vi "FGV_OEE_reference_selector.vi"(7 "options":T1, 8 "error_in":errorcluster, 11 "input":variant) -> (0 "error_out":errorcluster, 3 "output":variant)   [LabVIEW 2019]
uses:
  FGV_OEE_reference_selector.ctl
  OEE_reference_selecotr_references.ctl
  _misc/AULocalize/SubVIs/Get Localized Phrase Compact Interface 0D.vi
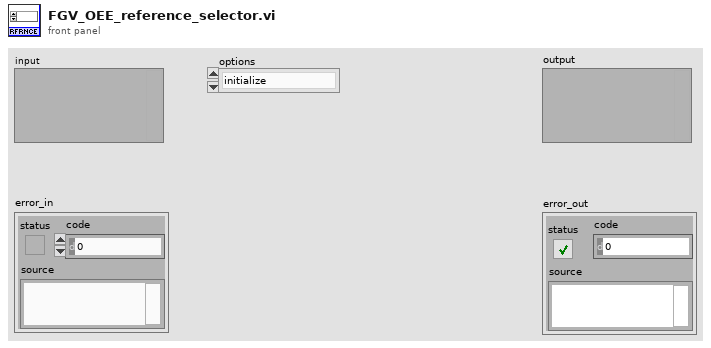
[diagram p1: front panel]
types:
  T1 = typedef "FGV_OEE_reference_selector.ctl" = enum16{"initialize", "set_values", "enable", "disable", "disable_gray", "get_reference_list", "get_active_reference"}
  T2 = typedef "OEE_reference_selecotr_references.ctl" = cluster{"reference_list":string[], "reference_selector":refnum<vi>, "reload_reference_list":refnum<vi>, "toggle_pulses":refnum<vi>}
  T3 = enum8{"Enabled", "Disabled", "Disabled and Grayed Out"}
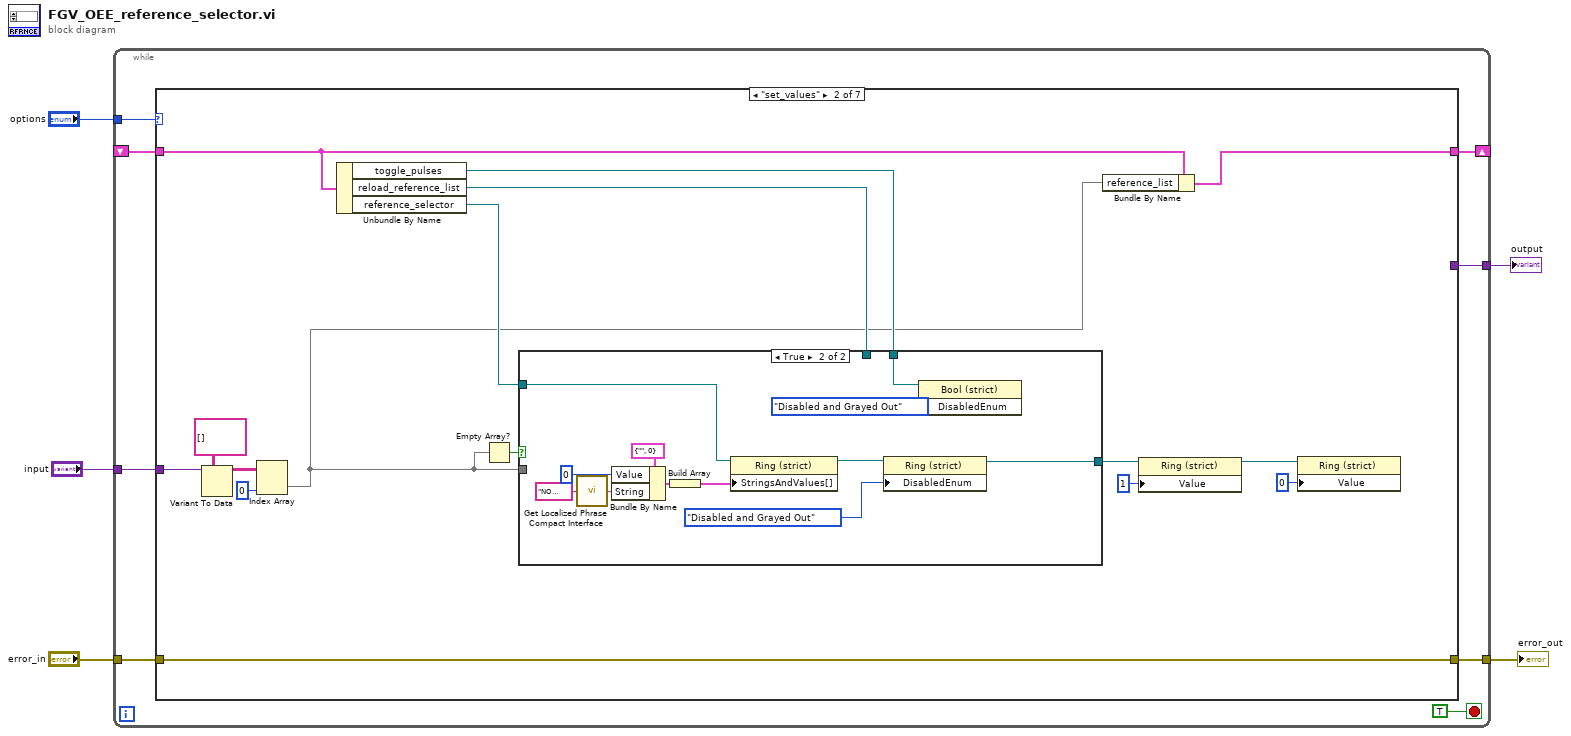
[diagram p0: block diagram]
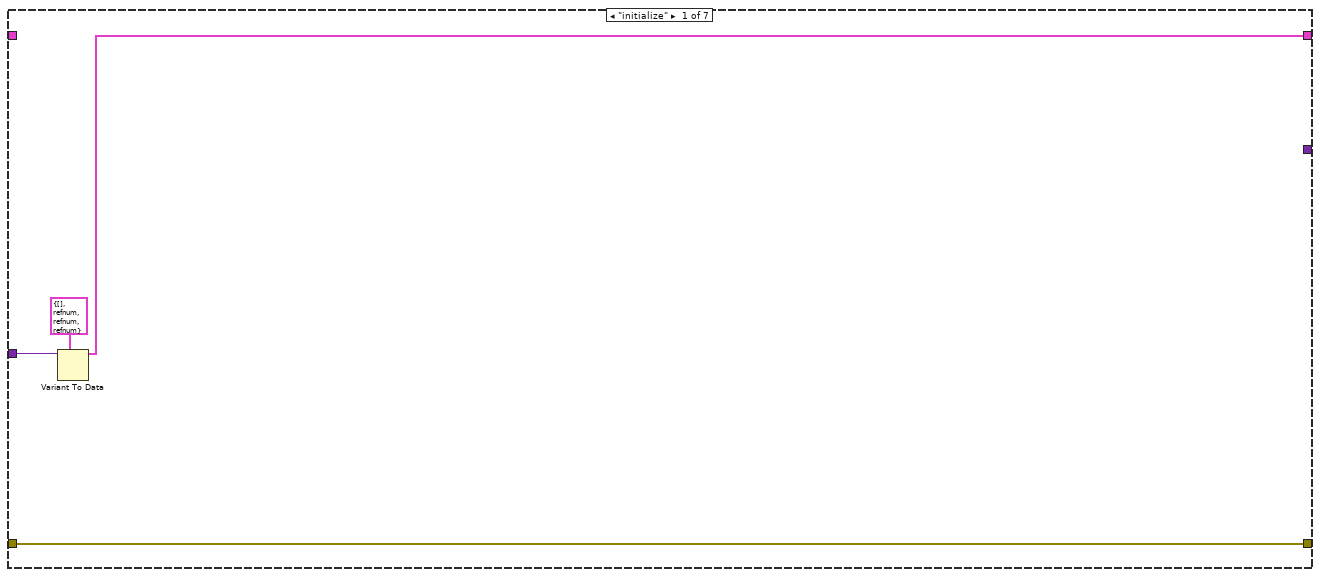
[diagram p2: hidden frame]
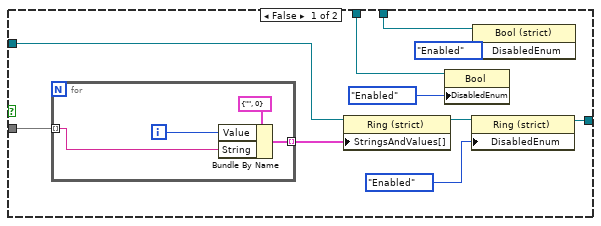
[diagram p3: hidden frame]
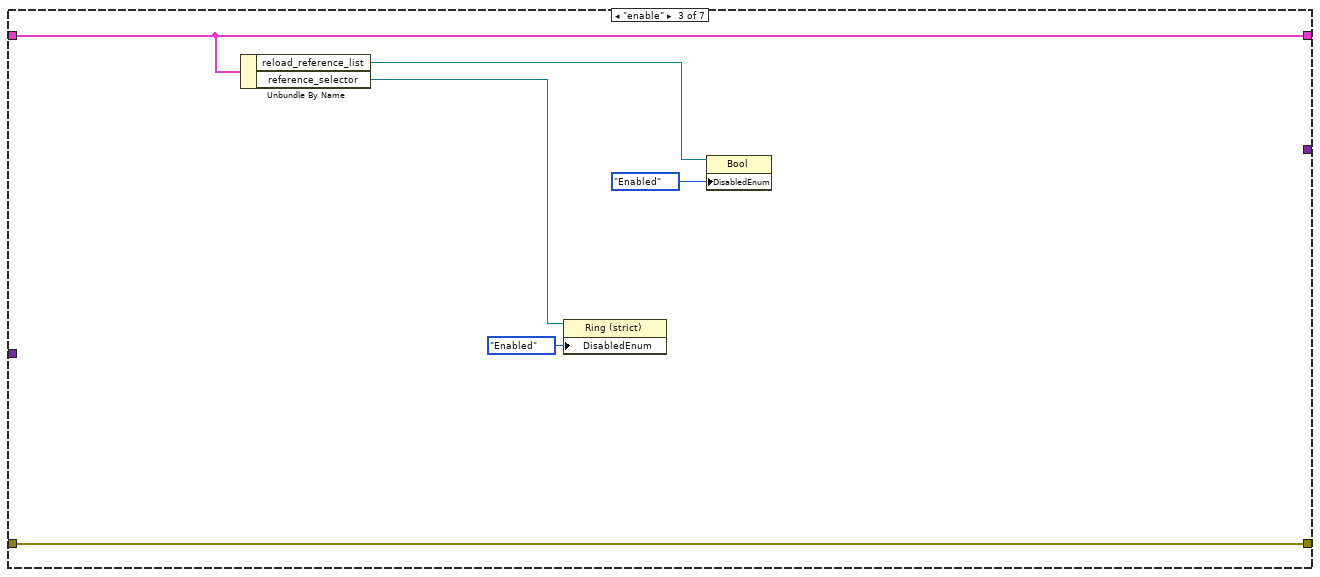
[diagram p4: hidden frame]
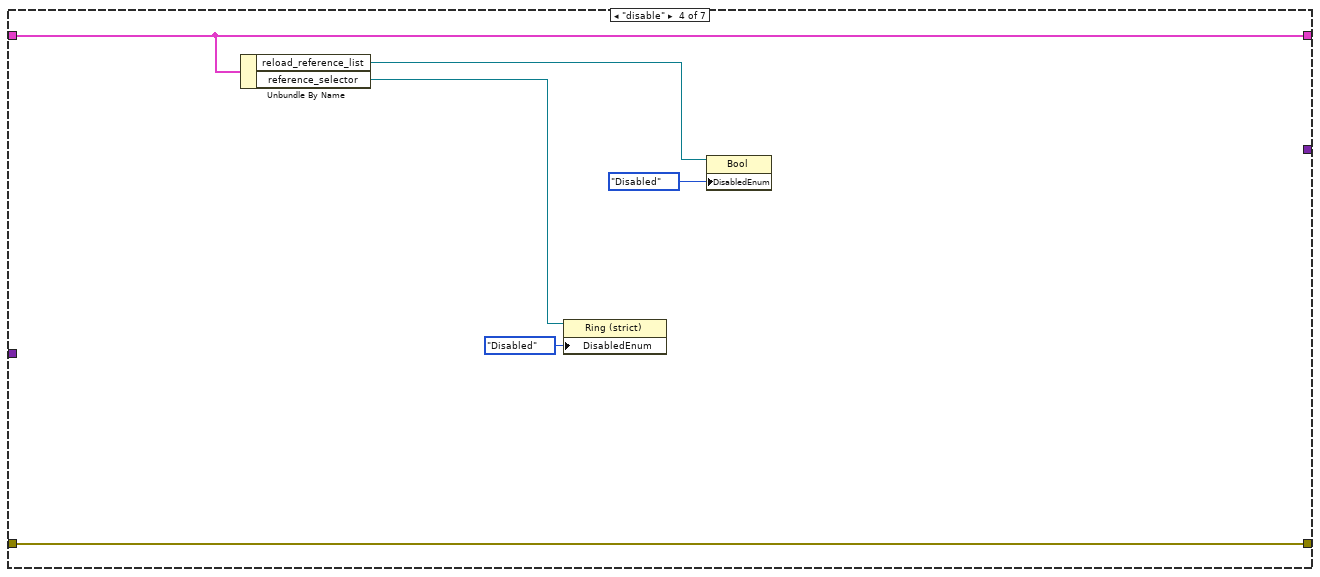
[diagram p5: hidden frame]
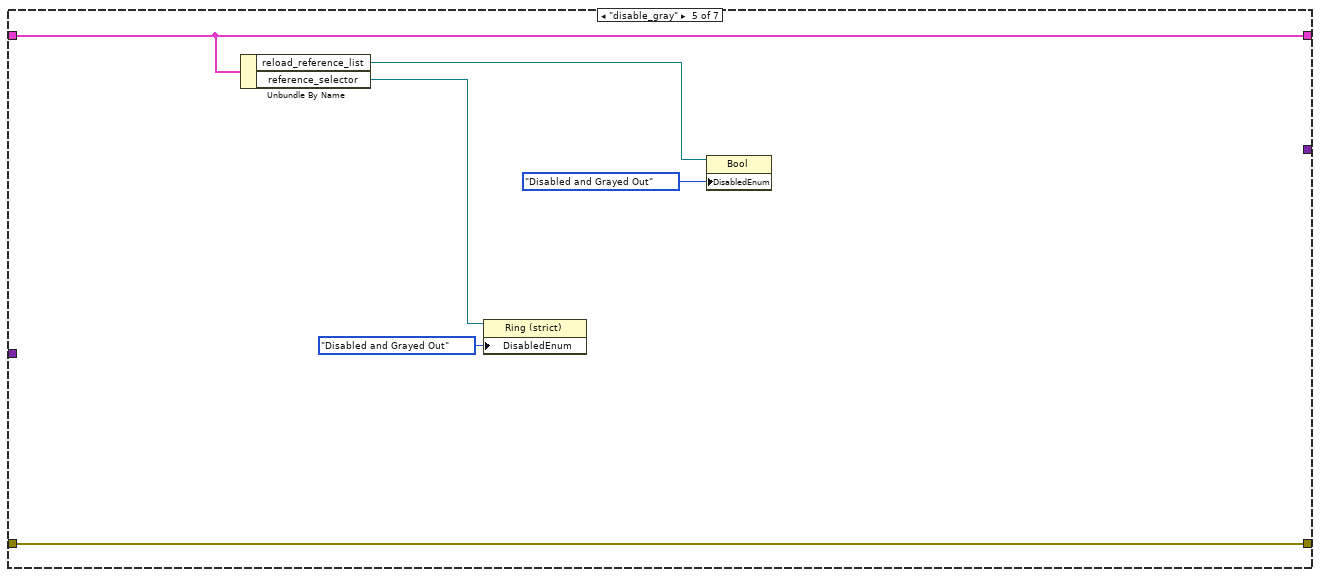
[diagram p6: hidden frame]
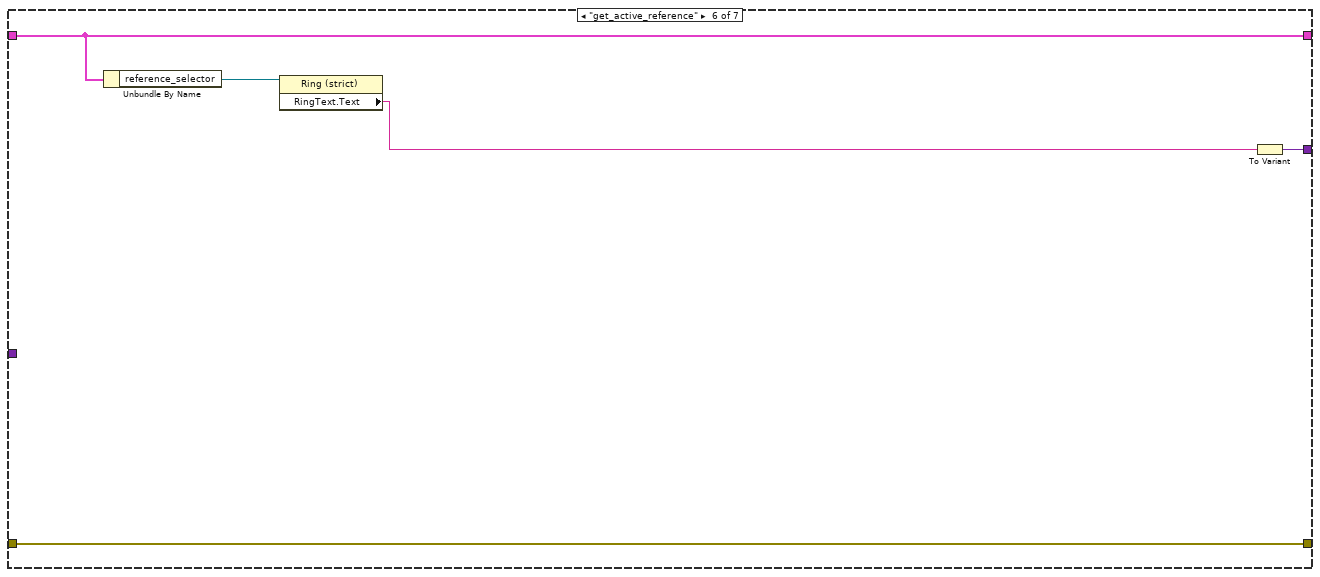
[diagram p7: hidden frame]
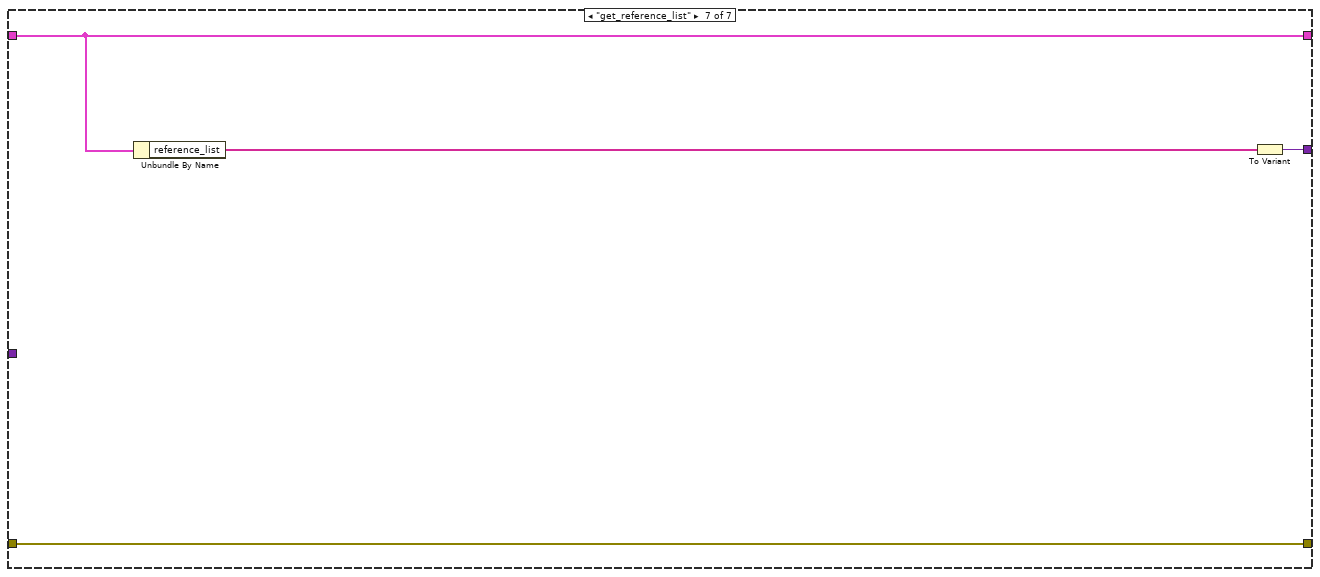
[diagram p8: hidden frame]
diagram:
  n1 = while {
    tunnel: "options" -> [w12]
    tunnel: [w11] -> w5
    tunnel: "error_in" -> [w10]
    shift-right: [w9] -> _
    shift-left: _ -> [w8]
    tunnel: "input" -> [w7]
    tunnel: [w6] -> w1
    stop <- TRUE stop-if-true
    n2 = case shown="\"set_values\"" w12 {
      tunnel: [w17 w33 w65 w71 w77 w82 w86] -> w11
      tunnel: w10 -> [w17 w33 w65 w71 w77 w82 w86]
      tunnel: [w14 w19 w62 w68 w74 w80 w84] -> w9
      tunnel: w8 -> [_ w20 w62 w68 w74 w80 w84]
      tunnel: w7 -> [w16 w32 _ _ _ _ _]
      tunnel: [_ _ _ _ _ w81 w85] -> w6
      frame "initialize" {
        n3 = Variant To Data(type=T2 {"reference_list"=[], "reference_selector"=refnum, "reload_reference_list"=refnum, "toggle_pulses"=refnum} ("OBJ_references"), Variant=w16) -> (data=w14:T2)  [unwired: 1 in, 1 out]
      }
      frame "set_values" {
        n4 = Variant To Data(type=string[][] [] ("strings"), Variant=w32) -> (data=w25:string[][])  [unwired: 1 in, 1 out]
        n5 = Index Array(array=w25, index (col)=0 ("index (row)")) -> (element=w18:string[])  [unwired: 1 in]
        n6 = Unbundle By Name(w20) -> ("toggle_pulses"=w21:refnum<vi>, "reload_reference_list"=w22:refnum<vi>, "reference_selector"=w23:refnum<vi>)
        n7 = Empty Array?(array=w18) -> (empty?=w26:bool)
        n8 = case shown="True" w26 {
          tunnel: w23 -> [w43 w54]
          tunnel: w18 -> [w38 _]
          tunnel: [w41 w51] -> w28
          tunnel: w22 -> [w36 _]
          tunnel: w21 -> [w35 w50]
          frame False {
            n9 = for {
              tunnel: w38 -> [w44] mode=indexing
              tunnel: [w46] -> w39 mode=indexing
              i -> [w45]
              n10 = Bundle By Name(cluster=cluster{"String":string, "Value":u16} {"String"="", "Value"=0}, "Value"=w45, "String"=w44) -> (w46:cluster{"String":string, "Value":u16})
            }
            n11 = property class="Ring (strict)"(reference=w43, "StringsAndValues[]"=w39) -> (reference out=w42:refnum<vi>)  [unwired: 1 in, 1 out]
            n12 = property class="Bool"(reference=w36, "DisabledEnum"=T3."Enabled" ("Disabled")) -> ()  [unwired: 1 in, 2 out]
            n13 = property class="Ring (strict)"(reference=w42, "DisabledEnum"=T3."Enabled" ("Disabled")) -> (reference out=w41:refnum<vi>)  [unwired: 1 in, 1 out]
            n14 = property class="Bool (strict)"(reference=w35, "DisabledEnum"=T3."Enabled" ("Disabled")) -> ()  [unwired: 1 in, 2 out]
          }
          frame True {
            n15 = call-poly "Get Localized Phrase Compact Interface.vi"("Key"="NO VALID REFERENCE FOUND" ("String")) -> ("Translated Phrase"=w48:string)
            n16 = Bundle By Name(cluster=cluster{"String":string, "Value":u16} {"String"="", "Value"=0}, "Value"=u16 0, "String"=w48) -> (w55:cluster{"String":string, "Value":u16})
            n17 = Build Array(w55) -> (w56:cluster{"String":string, "Value":u16}[])
            n18 = property class="Ring (strict)"(reference=w54, "StringsAndValues[]"=w56) -> (reference out=w53:refnum<vi>)  [unwired: 1 in, 1 out]
            n19 = property class="Ring (strict)"(reference=w53, "DisabledEnum"=T3."Disabled and Grayed Out" ("Disabled")) -> (reference out=w51:refnum<vi>)  [unwired: 1 in, 1 out]
            n20 = property class="Bool (strict)"(reference=w50, "DisabledEnum"=T3."Disabled and Grayed Out" ("Disabled")) -> ()  [unwired: 1 in, 2 out]
          }
        }
        n21 = Bundle By Name(cluster=w20, "reference_list"=w18) -> (w19:T2)
        n22 = property class="Ring (strict)"(reference=w28, "Value"=u16 1) -> (reference out=w27:refnum<vi>)  [unwired: 1 in, 1 out]
        n23 = property class="Ring (strict)"(reference=w27, "Value"=u16 0) -> ()  [unwired: 1 in, 2 out]
      }
      frame "enable" {
        n24 = Unbundle By Name(w62) -> ("reload_reference_list"=w60:refnum<vi>, "reference_selector"=w61:refnum<vi>)
        n25 = property class="Ring (strict)"(reference=w61, "DisabledEnum"=T3."Enabled" ("Disabled")) -> ()  [unwired: 1 in, 2 out]
        n26 = property class="Bool"(reference=w60, "DisabledEnum"=T3."Enabled" ("Disabled")) -> ()  [unwired: 1 in, 2 out]
      }
      frame "disable" {
        n27 = Unbundle By Name(w68) -> ("reload_reference_list"=w66:refnum<vi>, "reference_selector"=w67:refnum<vi>)
        n28 = property class="Ring (strict)"(reference=w67, "DisabledEnum"=T3."Disabled" ("Disabled")) -> ()  [unwired: 1 in, 2 out]
        n29 = property class="Bool"(reference=w66, "DisabledEnum"=T3."Disabled" ("Disabled")) -> ()  [unwired: 1 in, 2 out]
      }
      frame "disable_gray" {
        n30 = Unbundle By Name(w74) -> ("reload_reference_list"=w72:refnum<vi>, "reference_selector"=w73:refnum<vi>)
        n31 = property class="Ring (strict)"(reference=w73, "DisabledEnum"=T3."Disabled and Grayed Out" ("Disabled")) -> ()  [unwired: 1 in, 2 out]
        n32 = property class="Bool"(reference=w72, "DisabledEnum"=T3."Disabled and Grayed Out" ("Disabled")) -> ()  [unwired: 1 in, 2 out]
      }
      frame "get_active_reference" {
        n33 = Unbundle By Name(w80) -> ("reference_selector"=w79:refnum<vi>)
        n34 = property class="Ring (strict)"(reference=w79) -> ("RingText.Text"=w78:string)  [unwired: 1 in, 2 out]
        n35 = To Variant(anything=w78) -> (Variant=w81:variant)
      }
      frame "get_reference_list" {
        n36 = Unbundle By Name(w84) -> ("reference_list"=w83:string[])
        n37 = To Variant(anything=w83) -> (Variant=w85:variant)
      }
    }
  }
  "error_out" <- w5
  "output" <- w1
